vi "Initialize Configuration VI.vi"(4 "Step Number":i32, 6 "Step Name":string, 8 "error in (no error)":errorcluster, 10 "Subpanel Queue in":refnum<queue>, 11 "Configured Steps In":T1[](array[typedef])) -> (0 "error out":errorcluster, 2 "VI Reference out":T2, 3 "Configured Steps Out":T1[](array[typedef]))   [LabVIEW 2018]
doc: "This VI starts the configuration VI associated with the currently selected control step in the 'Control Sequence' listbox. If the selected step has been configured, the existing configuration parameters are passed in as an input to the configuration VI. The queue is used to pass messages to the configuration VI."
uses:
  controls/VI Reference Type.ctl
  controls/Configured Step.ctl
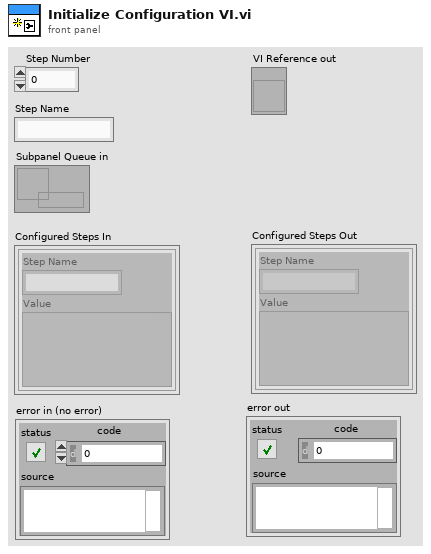
[diagram p1: front panel]
types:
  T1 = typedef "Configured Step.ctl" = cluster{"Step Name":string, "Value":variant}
  T2 = typedef "VI Reference Type.ctl" = refnum<vi>
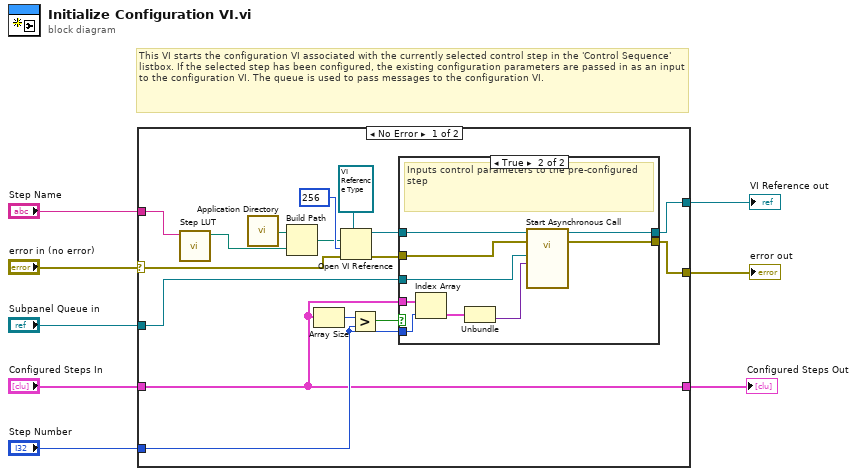
[diagram p0: block diagram]
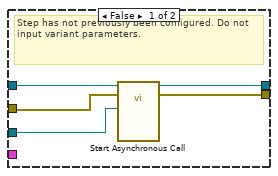
[diagram p2: hidden frame]
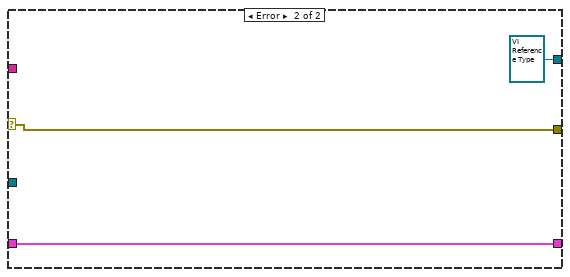
[diagram p3: hidden frame]
diagram:
  # "This VI starts the configuration VI associated with the currently selected control step in the 'Control Sequence' listbox. If the selected step has been configured, the existing configuration parameters are passed in as an input to the configuration VI. The queue is used to pass messages to the configuration VI."
  n1 = case shown="No Error" "error in (no error)" {
    selector: "error in (no error)" -> [w10 w40]
    tunnel: "Subpanel Queue in" -> [w23 _]
    tunnel: [w20 T2 refnum ("VI reference")] -> w7
    tunnel: "Step Number" -> [w18 _]
    tunnel: "Configured Steps In" -> [w9 w39]
    tunnel: [w15 w40] -> w4
    tunnel: "Step Name" -> [w12 _]
    tunnel: [w9 w39] -> w1
    frame No Error {
      n2 = call "Step LUT.vi"("Step Name"=w12) -> ("Relative Path"=w14:path)  [unwired: 9 in, 1 out]
      n3 = call <vilib>:"Application Directory.vi"() -> ("Application Directory"=w11:path)
      n4 = Build Path(base path=w11, name or relative path=w14) -> (appended path=w13:path)
      n5 = Array Size(array=w9) -> (size(s)=w17:i32)
      n6 = Open VI Reference(type specifier VI Refnum (for type only)=T2 refnum ("VI reference"), vi path=w13, options=256, error in (no error)=w10) -> (vi reference=w21:T2, error out=w22:errorcluster)  [unwired: 2 in]
      n7 = Greater?(x=w17, y=w18) -> (0:w19:bool)
      n8 = case shown="True" w19 {
        tunnel: w9 -> [_ w38]
        tunnel: w18 -> [_ w37]
        tunnel: [w26 w31] -> w15
        tunnel: [w25 w30] -> w20
        tunnel: w21 -> [w28 w33]
        tunnel: w22 -> [w29 w34]
        tunnel: w23 -> [w27 w35]
        frame False {
          # "Step has not previously been configured. Do not input variant parameters."
          n9 = call-by-ref "Start Asynchronous Call"(reference=w28, error in=w29, "Queue In"=w27) -> (reference out=w25:T2, error out=w26:errorcluster)  [unwired: 9 in, 2 out]
        }
        frame True {
          # "Inputs control parameters to the pre-configured step"
          n10 = Index Array(array=w38, index=w37) -> (element=w36:T1)
          n11 = Unbundle(w36) -> ("Value"=w32:variant)  [unwired: 1 out]
          n12 = call-by-ref "Start Asynchronous Call"(reference=w33, error in=w34, "Parameters In"=w32, "Queue In"=w35) -> (reference out=w30:T2, error out=w31:errorcluster)  [unwired: 8 in, 2 out]
        }
      }
    }
    frame Error {
    }
  }
  "VI Reference out" <- w7
  "error out" <- w4
  "Configured Steps Out" <- w1
